vi "Control Read Char From File.vi"(1 "default name if empty":string, 4 "prompt":string, 5 "[pattern]":string, 6 "RT Remote File Storage":bool, 7 "RT reference":refnum<vi>, 8 "System Path":path, 9 "Connected to RT":bool, 10 "file path":path) -> (2 "character string":string, 3 "new file path (NotAPath if cancelled)":path)   [LabVIEW 2023]
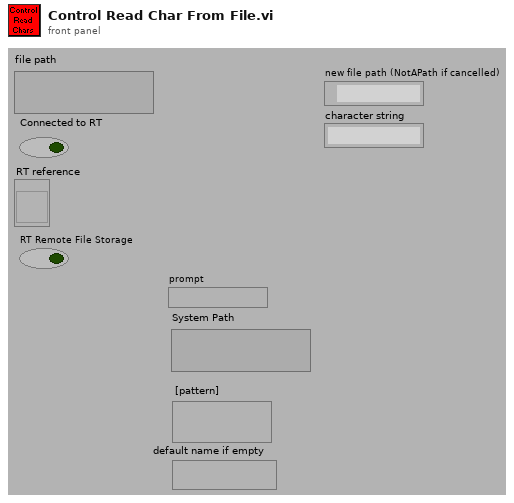
[diagram p1: front panel]
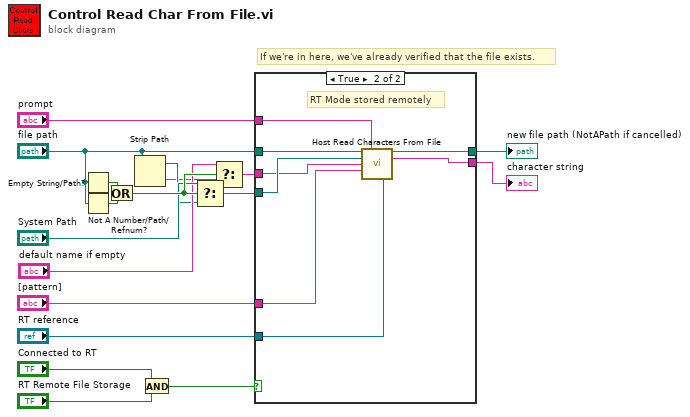
[diagram p0: block diagram]
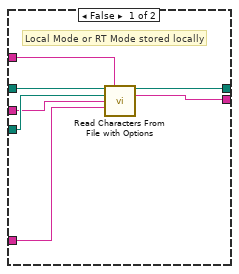
[diagram p2: hidden frame]
diagram:
  # "If we're in here, we've already verified that the file exists."
  n1 = Empty String/Path?(string/path="file path") -> (empty?=w11:bool)
  n2 = Not A Number/Path/Refnum?(number/path/refnum="file path") -> (NaN/Path/Refnum?=w10:bool)
  n3 = Or(x=w11, y=w10) -> (x .or. y?=w7:bool)
  n4 = Strip Path(path="file path") -> (stripped path=w3:path, name=w2:string)
  n5 = And(x="Connected to RT", y="RT Remote File Storage") -> (x .and. y?=w14:bool)
  n6 = Select(t="System Path", s=w7, f=w3) -> (s? t:f=w8:path)
  n7 = Select(t="default name if empty", s=w7, f=w2) -> (s? t:f=w6:string)
  n8 = case shown="True" w14 {
    tunnel: "RT reference" -> [_ w30]
    tunnel: [w24 w32] -> w18
    tunnel: [w23 w31] -> w17
    tunnel: "file path" -> [w25 w33]
    tunnel: "prompt" -> [w21 w29]
    tunnel: w8 -> [w22 w28]
    tunnel: w6 -> [w20 w27]
    tunnel: "[pattern]" -> [w19 w26]
    frame False {
      # "Local Mode or RT Mode stored locally"
      n9 = call "Read Characters From File with Options.vi"("file path (dialog if empty)"=w25, "prompt"=w21, "start path (Not A Path)"=w22, "default name"=w20, "[pattern]"=w19) -> ("new file path (NotAPath if cancelled)"=w24:path, "character string"=w23:string)  [unwired: 6 in, 3 out]
    }
    frame True {
      # "RT Mode stored remotely"
      n10 = call "Host Read Characters From File.vi"("file path"=w33, "prompt"=w29, "start path (Not A Path)"=w28, "default name"=w27, "[pattern]"=w26, "RT Reference"=w30) -> ("new file path (NotAPath if cancelled)"=w32:path, "character string"=w31:string)  [unwired: 5 in, 3 out]
    }
  }
  "new file path (NotAPath if cancelled)" <- w18
  "character string" <- w17
